vi "ADXRS453_Test.vi"() -> ()   [LabVIEW 2014]
uses:
  <vilib>/Rock Robotics/SystemInterfaces/spilib/spi_bus.ctl
  ADXRS453_Global.vi
panel:
  out "Gyro Angle":dbl(graph)
  out "Gyro Drift":dbl(graph)
  in  "Stop":bool
  out "Gyro Angle (degrees)":dbl
  out "Gyro Output (dps)":dbl
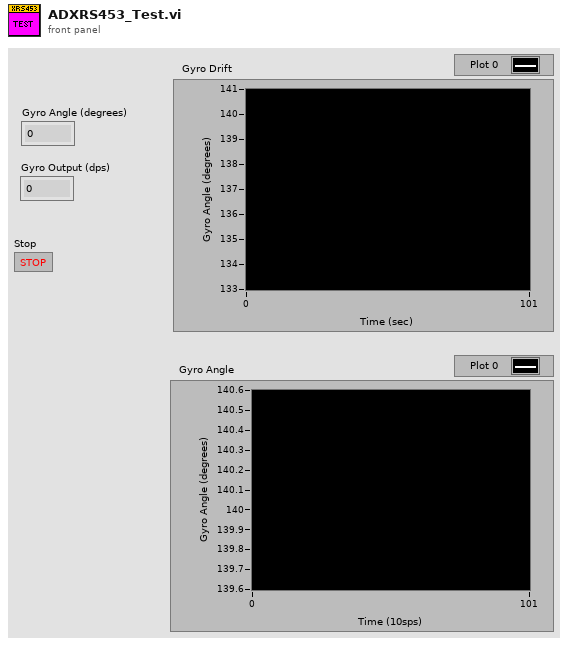
[diagram p1: front panel]
types:
  T1 = typedef "spi_bus.ctl" = enum16{"SPI On-Board, CS0", "SPI On-Board, CS1", "SPI On-Board, CS2", "SPI On-Board, CS3", "SPI MXP", "Invalid"}
  T2 = typedef "WPI_SPIDevRef.ctl" = cluster{"DevStatus":errorcluster, "Handle":i32, "Controller":T3, "SPI Bus":T1}
  T3 = typedef "FPGA_TypedefDigitalModule.ctl" = enum16{"Controller 1"}
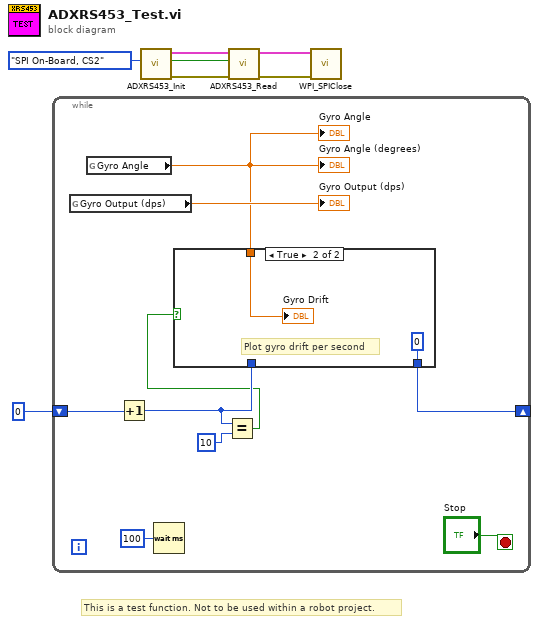
[diagram p0: block diagram]
diagram:
  # "This is a test function. Not to be used within a robot project."
  n1 = while {
    shift-right: [w11] -> _
    shift-left: 0 -> [w12]
    stop <- "Stop" stop-if-true
    n2 = global read "ADXRS453_Global.vi" "Gyro Output (dps)"() -> (→"Gyro Output (dps)":dbl)
    n3 = global read "ADXRS453_Global.vi" "Gyro Angle"() -> (w8:dbl)
    "Gyro Angle (degrees)" <- w8
    "Gyro Angle" <- w8
    n4 = Increment(x=w12) -> (x+1=w10:i32)
    n5 = Wait (ms)(milliseconds to wait=u32 100) -> ()  [unwired: 1 out]
    n6 = Equal?(x=w10, y=10) -> (x = y?=w9:bool)
    n7 = case shown="True" w9 {
      tunnel: w8 -> [_ w19]
      tunnel: [w17 0] -> w11
      tunnel: w10 -> [w17 _]
      frame False {
      }
      frame True {
        # "Plot gyro drift per second"
        "Gyro Drift" <- w19
      }
    }
  }
  n8 = call "ADXRS453_Init.vi"("SPI Bus"=spi_bus."SPI On-Board, CS2") -> ("Error Out"=w6:errorcluster, "Gyro Detected?"=w5:bool, "ADXRS453 Ref Out"=w7:T2)  [unwired: 8 in]
  n9 = call "ADXRS453_Read.vi"("Error In"=w6, "Gyro Detected?"=w5, "ADXRS453 Ref In"=w7) -> ("Error Out"=w3:errorcluster, "ADXRS453 Ref Out"=w2:T2)  [unwired: 7 in]
  n10 = call <vilib>:"WPI_SPIClose.vi"("error in (no error)"=w3, "SPIDevRef"=w2) -> ()  [unwired: 9 in, 1 out]
